vi "EndienSwap.vi"(11 "name (unnamed)":string) -> (3 "concatenated string":string)   [LabVIEW 2012]
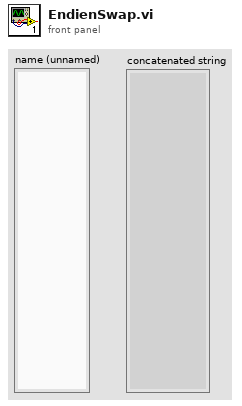
[diagram p1: front panel]
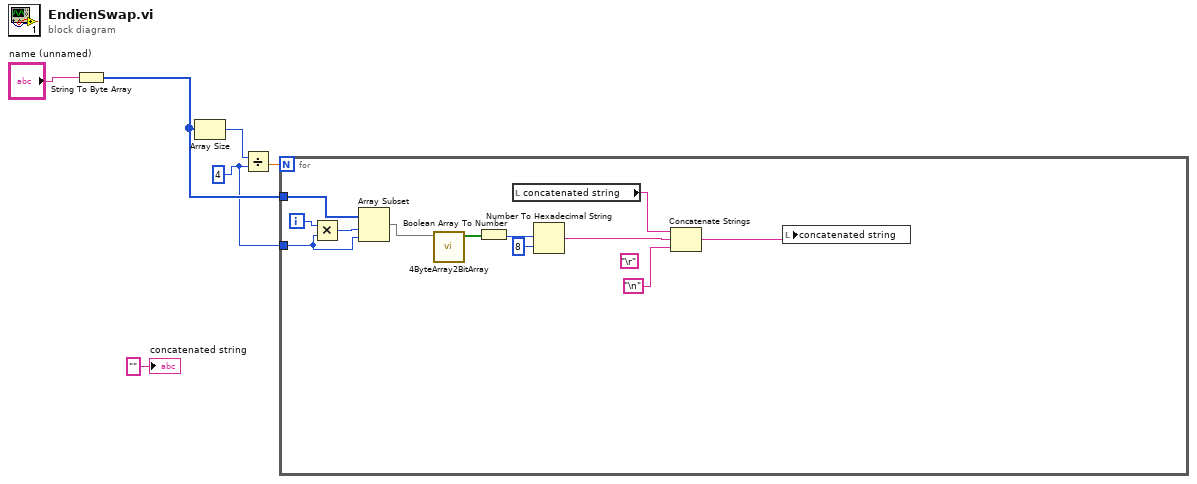
[diagram p0: block diagram]
diagram:
  w3 = 4 ("y")
  n1 = String To Byte Array(string="name (unnamed)") -> (unsigned byte array=w5:u8[])
  n2 = Array Size(array=w5) -> (size(s)=w2:i32)
  n3 = Divide(x=w2, y=w3) -> (x/y=w4:dbl)
  n4 = for {
    N: w4 -> [_]
    tunnel: w5 -> [w18]
    tunnel: w3 -> [w14]
    i -> [w16]
    (unwired) "\r"
    n5 = Multiply(x=w16, y=w14) -> (x*y=w17:i32)
    n6 = Array Subset(array=w18, index=w17, length=w14) -> (w15:u8[])
    n7 = call "4ByteArray2BitArray.vi"("array"=w15) -> ("Array"=w11:bool[])  [unwired: 10 in]
    n8 = Boolean Array To Number(Boolean array=w11) -> (number=w12:u32)
    n9 = local read "concatenated string"() -> (w9:string)
    n10 = Number To Hexadecimal String(1:i16 8 ("width (-)"), 2:w12) -> (0:w10:string)
    n11 = Concatenate Strings(w9, w10, "\n") -> (w8:string)
    n12 = local write "concatenated string"(w8) -> ()
  }
  "concatenated string" <- "" ("concatenated string")
